vi "Create Channel Task.vi"(8 "error in (no error)":errorcluster, 11 "DI in":refnum<class "DI.lvclass">) -> (0 "error out":errorcluster, 3 "DI out":refnum<class "DI.lvclass">)   [LabVIEW 2023, in "HardwareAbstractionLayer_LVOOP.lvlib" / "DI.lvclass"]
uses:
  DI.lvclass
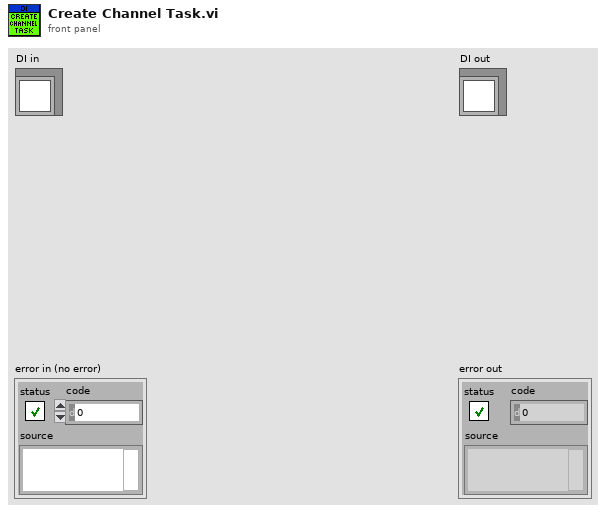
[diagram p1: front panel]
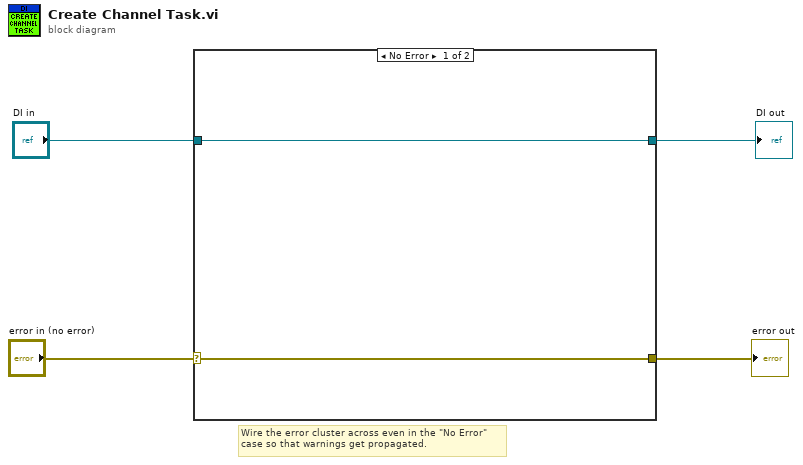
[diagram p0: block diagram]
diagram:
  # "Wire the error cluster across even in the \"No Error\"\ncase so that warnings get propagated."
  n1 = case shown="No Error" "error in (no error)" {
    selector: "error in (no error)" -> [w5 w8]
    tunnel: [w5 w8] -> w3
    tunnel: [w6 w7] -> w1
    tunnel: "DI in" -> [w6 w7]
    frame No Error {
    }
    frame Error {
    }
  }
  "error out" <- w3
  "DI out" <- w1
